vi "YAG_init.v4.vi"(8 "error in (no error)":errorcluster, 9 "initial V":dbl=700.0, 10 "initial rep rate":dbl=10.0, 11 "VISA Refnum in":refnum<visa-resource-name>="COM1") -> (0 "error out":errorcluster={"status"=FALSE, "code"=1073676294, "source"="VISA Read in Cmd-Reply.vi->YAG_init.vi->YAG_Control.v2.vi"}, 3 "VISA Refnum out":refnum<visa-resource-name>="COM1")   [LabVIEW 2018]
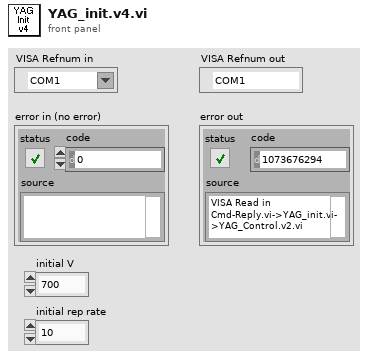
[diagram p1: front panel]
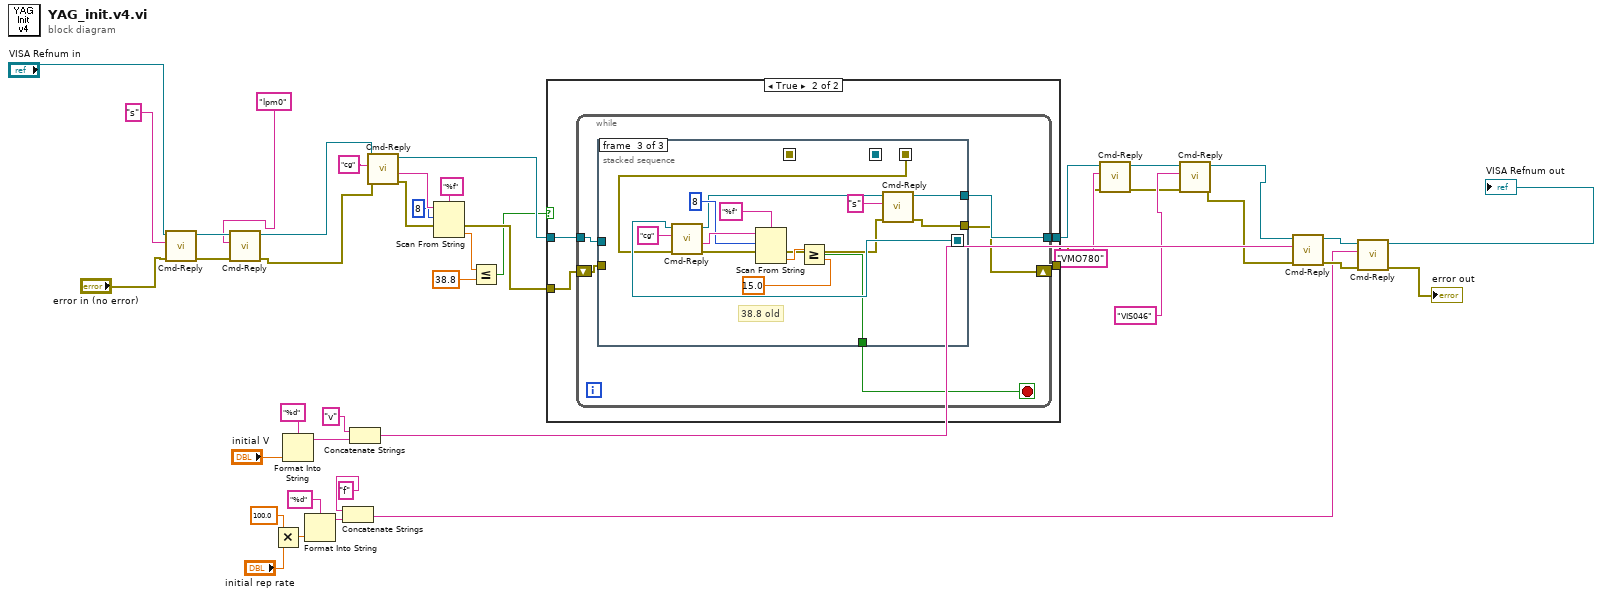
[diagram p0: block diagram]
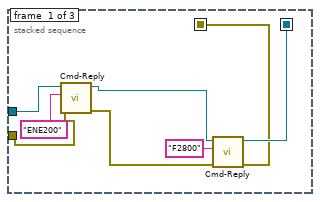
[diagram p3: hidden frame]
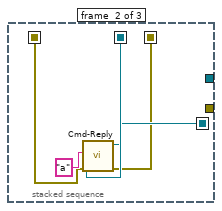
[diagram p4: hidden frame]
diagram:
  n1 = call "Cmd-Reply.vi"("error in (no error)"="error in (no error)", "cmd"="s", "VISA Refnum in"="VISA Refnum in") -> ("error out"=w39:errorcluster, "VISA Refnum out"=w38:refnum<visa-resource-name>)  [unwired: 6 in, 1 out]
  n2 = call "Cmd-Reply.vi"("error in (no error)"=w39, "cmd"="lpm0", "VISA Refnum in"=w38) -> ("error out"=w13:errorcluster, "VISA Refnum out"=w15:refnum<visa-resource-name>)  [unwired: 6 in, 1 out]
  n3 = Multiply(x=100.0, y="initial rep rate") -> (x*y=w31:dbl)
  n4 = Format Into String(format string="%d", "initial V") -> (resulting string=w36:string)  [unwired: 2 in, 1 out]
  n5 = Format Into String(format string="%d", w31) -> (resulting string=w29:string)  [unwired: 2 in, 1 out]
  n6 = Concatenate Strings("f" ("string"), w29) -> (w23:string)
  n7 = Concatenate Strings("v" ("string"), w36) -> (w21:string)
  n8 = call "Cmd-Reply.vi"("error in (no error)"=w13, "cmd"="cg" ("write buffer"), "VISA Refnum in"=w15) -> ("error out"=w17:errorcluster, "reply"=w19:string, "VISA Refnum out"=w14:refnum<visa-resource-name>)  [unwired: 6 in]
  n9 = Scan From String(format string="%f", input string=w19, initial scan location=u32 8, error in=w17) -> (error out=w12:errorcluster, output 1=w11:dbl)  [unwired: 1 in, 2 out]
  n10 = Less Or Equal?(x=w11, y=38.8) -> (x <= y?=w9:bool)
  n11 = case shown="True" w9 {
    tunnel: w14 -> [w44 w48]
    tunnel: [w44 w45] -> w4
    tunnel: w12 -> [w43 w47]
    tunnel: [w43 w46] -> w2
    frame False {
    }
    frame True {
      n12 = while {
        tunnel: w48 -> [w53]
        shift-right: [w49] -> w46
        shift-left: w47 -> [w51]
        tunnel: [w50] -> w45
        stop <- w52 stop-if-true
        n13 = stacked-sequence {
          seq-local: [w57 _ _] -> [_ w66 _]
          seq-local: [_ w65 _] -> [_ _ w74]
          seq-local: [w55 _ _] -> [_ w63 _]
          seq-local: [_ w62 _] -> [_ _ w72]
          tunnel: w53 -> [w61 _ _]
          tunnel: [_ _ w73] -> w52
          tunnel: w51 -> [w59 _ _]
          tunnel: [_ _ w69] -> w50
          tunnel: [_ _ w67] -> w49
          frame #0 {
            n14 = call "Cmd-Reply.vi"("error in (no error)"=w59, "cmd"="ENE200", "VISA Refnum in"=w61) -> ("error out"=w56:errorcluster, "VISA Refnum out"=w58:refnum<visa-resource-name>)  [unwired: 6 in, 1 out]
            n15 = call "Cmd-Reply.vi"("error in (no error)"=w56, "cmd"="F2800", "VISA Refnum in"=w58) -> ("error out"=w55:errorcluster, "VISA Refnum out"=w57:refnum<visa-resource-name>)  [unwired: 6 in, 1 out]
          }
          frame #1 {
            n16 = call "Cmd-Reply.vi"("error in (no error)"=w63, "cmd"="a", "VISA Refnum in"=w66) -> ("error out"=w62:errorcluster, "VISA Refnum out"=w65:refnum<visa-resource-name>)  [unwired: 6 in, 1 out]
          }
          frame #2 {
            # "38.8 old"
            n17 = call "Cmd-Reply.vi"("error in (no error)"=w72, "cmd"="cg" ("write buffer"), "VISA Refnum in"=w74) -> ("error out"=w78:errorcluster, "reply"=w80:string, "VISA Refnum out"=w70:refnum<visa-resource-name>)  [unwired: 6 in]
            n18 = Scan From String(format string="%f", input string=w80, initial scan location=u32 8, error in=w78) -> (error out=w68:errorcluster, output 1=w76:dbl)  [unwired: 1 in, 2 out]
            n19 = Greater Or Equal?(x=w76, y=15.0) -> (x >= y?=w73:bool)
            n20 = call "Cmd-Reply.vi"("error in (no error)"=w68, "cmd"="s", "VISA Refnum in"=w70) -> ("error out"=w67:errorcluster, "VISA Refnum out"=w69:refnum<visa-resource-name>)  [unwired: 6 in, 1 out]
          }
        }
      }
    }
  }
  n21 = call "Cmd-Reply.vi"("error in (no error)"=w2, "cmd"="VMO780" ("concatenated string"), "VISA Refnum in"=w4) -> ("error out"=w5:errorcluster, "VISA Refnum out"=w8:refnum<visa-resource-name>)  [unwired: 6 in, 1 out]
  n22 = call "Cmd-Reply.vi"("error in (no error)"=w5, "cmd"="VIS046" ("concatenated string"), "VISA Refnum in"=w8) -> ("error out"=w1:errorcluster, "VISA Refnum out"=w3:refnum<visa-resource-name>)  [unwired: 6 in, 1 out]
  n23 = call "Cmd-Reply.vi"("error in (no error)"=w1, "cmd"=w21, "VISA Refnum in"=w3) -> ("error out"=w25:errorcluster, "VISA Refnum out"=w27:refnum<visa-resource-name>)  [unwired: 6 in, 1 out]
  n24 = call "Cmd-Reply.vi"("error in (no error)"=w25, "cmd"=w23, "VISA Refnum in"=w27) -> ("error out"=→"error out":errorcluster, "VISA Refnum out"=→"VISA Refnum out":refnum<visa-resource-name>)  [unwired: 6 in, 1 out]
